vi "Git Check whether Branch exists.vi"(8 "error in (no error)":errorcluster, 10 "DailyPatchBranchName":string, 11 "Path":path) -> (0 "error out":errorcluster, 2 "Boolean":bool)   [LabVIEW 2017]
doc: "lvAPT-User-Libraries 2022.4.27.213228\nYAO - lvAPT\nCopyright (c) 2022, lvAPT"
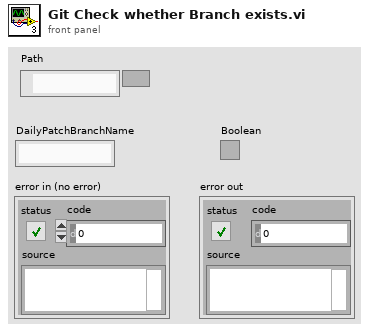
[diagram p1: front panel]
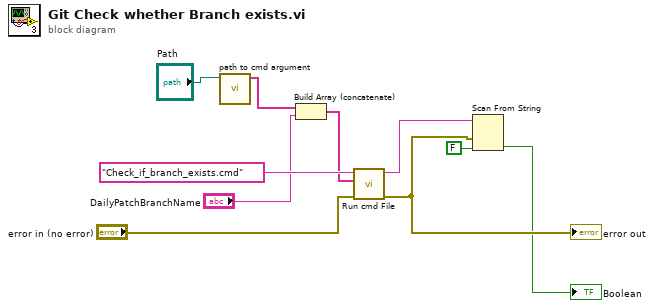
[diagram p0: block diagram]
diagram:
  n1 = call "path to cmd argument.vi"("path"="Path") -> ("Array"=w1:string[])  [unwired: 10 in]
  n2 = Build Array (concatenate)(w1, "DailyPatchBranchName") -> (w4:string[])
  n3 = call "Run cmd File.vi"("Error in"="error in (no error)", "args"=w4, "name or relative path"="Check_if_branch_exists.cmd") -> ("Error out"=w6:errorcluster, "standard output"=w7:string)  [unwired: 6 in, 1 out]
  "error out" <- w6
  n4 = Scan From String(input string=w7, error in=w6, default 1=FALSE) -> (output 1=→"Boolean":bool)  [unwired: 2 in, 3 out]
